vi "Noise_Out_A.vi"(2 "pico inalcanzable":dbl, 3 "IN":dbl(slide) scale=0.0..9000.0) -> (0 "cluster":cluster{"[0]":dbl, "[1]":dbl}, 1 "OUT":u32)   [LabVIEW 2017]
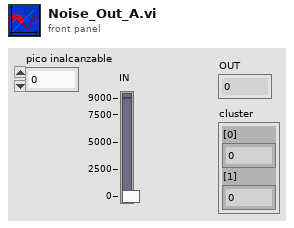
[diagram p1: front panel]
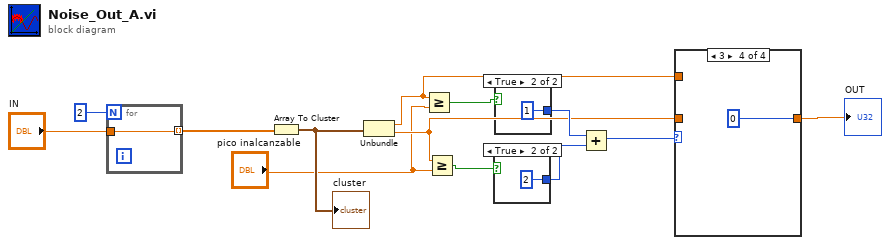
[diagram p0: block diagram]
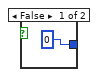
[diagram p5: hidden frame]
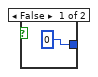
[diagram p6: hidden frame]
diagram:
  n1 = for {
    N: 2 -> [_]
    tunnel: [w14] -> w2 mode=indexing
    tunnel: "IN" -> [w14]
  }
  n2 = Array To Cluster(array=w2) -> (cluster=w13:cluster{"[0]":dbl, "[1]":dbl})
  "cluster" <- w13
  n3 = Unbundle(w13) -> ("[0]"=w6:dbl, "[1]"=w5:dbl)
  n4 = Greater Or Equal?(x=w6, y="pico inalcanzable") -> (x >= y?=w11:bool)
  n5 = Greater Or Equal?(x=w5, y="pico inalcanzable") -> (x >= y?=w12:bool)
  n6 = case shown="True" w12 {
    tunnel: [0 2] -> w9
    frame False {
    }
    frame True {
    }
  }
  n7 = case shown="True" w11 {
    tunnel: [0 1] -> w10
    frame False {
    }
    frame True {
    }
  }
  n8 = Add(x=w10, y=w9) -> (x+y=w8:i32)
  n9 = case shown="3" w8 {
    tunnel: [w19 w20 w21 0] -> w7
    tunnel: w6 -> [_ _ w21 _]
    tunnel: w5 -> [w19 w20 _ _]
    frame 0, Default {
    }
    frame 1 {
    }
    frame 2 {
    }
    frame 3 {
    }
  }
  "OUT" <- w7
